vi "onProcessStart.vi"(8 "error in (no error)":errorcluster, 11 "SystemController":refnum<class "SystemController.lvclass">) -> (0 "error out":errorcluster, 3 "SystemController out":refnum<class "SystemController.lvclass">)   [LabVIEW 2017, in "SystemController.lvclass"]
doc: "JKI State Machine Objects (SMO) 1.3.0.56\nJKI - JKI\nCopyright (c) 2017, JKI"
uses:
  SystemController.lvclass
  Camera/Camera_IMAQdx_class/Camera_IMAQdx.lvclass
  C:/VIT/simpleImageProcessingExample/lv_src/Camera/Camera_class/Camera.lvclass
  Camera/Camera_Sim_class/Camera_Sim.lvclass
  <vilib>/JKI/JKI SMO/SMO/SMO.lvclass
  ImageFacialDetection_class/ImageFacialDetection.lvclass
  Camera/Camera_class/Camera.lvclass
panel:
  # "For instructions on how to use the JKI State Machine Objects, examples and video tutorials, visit:\nhttp://jki.net/state-machine-objects/\n\nJKI State Machine Objects™\nhttp://jki.net/state-machine-objects/\nCopyright (C) 2005-2015, JKI <info@jki.net>\nALL RIGHTS RESERVED"
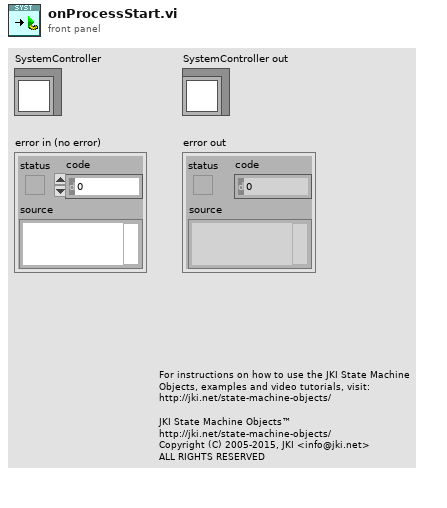
[diagram p1: front panel]
types:
  T1 = typedef "SystemController.lvclass/Configuration--Cluster.ctl" = cluster{"Camera":T2, "Find Eyes":bool, "Acquisition Rate (ms)":i32, "Image Buffer Length":i32}
  T2 = typedef "SystemController.lvclass/CameraConfig--Cluster.ctl" = cluster{"Simulate Camera":bool, "IMAQ Camera":T3, "Simulated Image Folder":path}
  T3 = typedef "Camera_IMAQdx.lvclass/Configuration--Cluster.ctl" = cluster{"Camera Interface Name":string, "Number of Buffers":u32, "Image Name":string, "Image Type":T4}
  T4 = typedef "Image Type" = u32
  T5 = cluster{"reference out":refnum<class "Camera.lvclass">, "reference out":refnum<class "ImageFacialDetection.lvclass">}
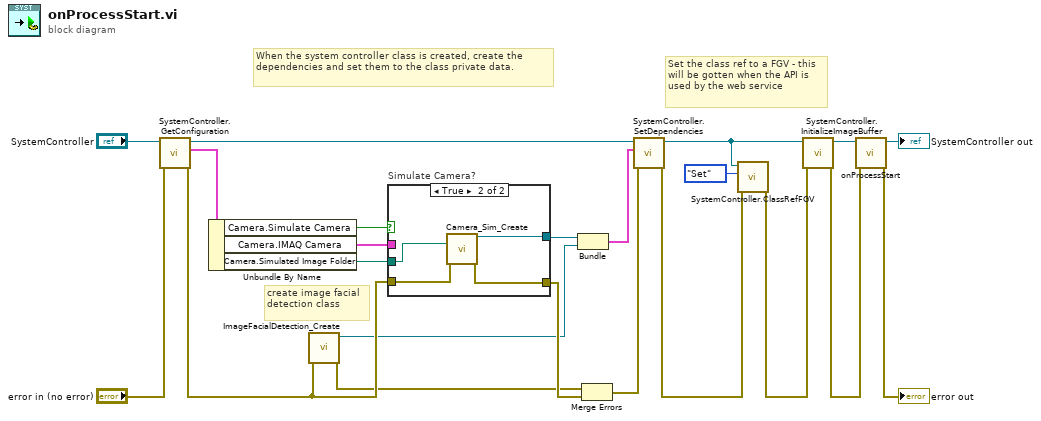
[diagram p0: block diagram]
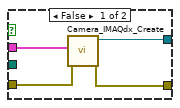
[diagram p2: hidden frame]
diagram:
  # "Set the class ref to a FGV - this will be gotten when the API is used by the web service"
  # "create image facial detection class"
  # "When the system controller class is created, create the dependencies and set them to the class private data."
  n1 = call "SystemController.GetConfiguration.vi"("error in (no error)"="error in (no error)", "SystemController"="SystemController") -> ("error out"=w10:errorcluster, "Configuration"=w17:T1, "SystemController out"=w19:refnum<class "SystemController.lvclass">)  [unwired: 7 in]
  n2 = Unbundle By Name(w17) -> ("Camera.Simulate Camera"=w16:bool, "Camera.IMAQ Camera"=w15:T3, "Camera.Simulated Image Folder"=w14:path)
  n3 = call "ImageFacialDetection_Create.vi"("error in (no error)"=w10) -> ("error out"=w8:errorcluster, "reference out"=w7:refnum<class "ImageFacialDetection.lvclass">)  [unwired: 9 in]
  n4 = case "Simulate Camera?" shown="True" w16 {
    tunnel: w15 -> [w26 _]
    tunnel: w14 -> [_ w30]
    tunnel: [w25 w29] -> w12
    tunnel: w10 -> [w24 w28]
    tunnel: [w23 w27] -> w13
    frame False {
      n5 = call "Camera_IMAQdx_Create.vi"("error in (no error)"=w24, "Configuration"=w26) -> ("error out"=w23:errorcluster, "reference out"=w25:refnum<class "Camera_IMAQdx.lvclass">)  [unwired: 8 in]
    }
    frame True {
      n6 = call "Camera_Sim_Create.vi"("Simulated Image Directory"=w30, "error in (no error)"=w28) -> ("reference out"=w29:refnum<class "Camera_Sim.lvclass">, "error out"=w27:errorcluster)  [unwired: 12 in]
    }
  }
  n7 = Bundle("reference out"=w12, "reference out"=w7) -> (w11:T5)  [unwired: 1 in]
  n8 = Merge Errors(w8, w13) -> (w9:errorcluster)
  n9 = call "SystemController.SetDependencies.vi"("error in (no error)"=w9, "Dependencies"=w11, "SystemController"=w19) -> ("error out"=w6:errorcluster, "SystemController out"=w4:refnum<class "SystemController.lvclass">)  [unwired: 7 in]
  n10 = call "SystemController.ClassRefFGV.vi"("error in (no error)"=w6, "Set/Get"=enum16{"Set", "Get"}."Set", "SystemController"=w4) -> ("error out"=w2:errorcluster)  [unwired: 7 in, 1 out]
  n11 = call "SystemController.InitializeImageBuffer.vi"("error in (no error)"=w2, "SystemController"=w4) -> ("error out"=w1:errorcluster, "SystemController out"=w3:refnum<class "SystemController.lvclass">)  [unwired: 8 in]
  n12 = call-parent "onProcessStart.vi"("error in (no error)"=w1, "SMO"=w3) -> ("error out"=→"error out":errorcluster, "SMO out"=→"SystemController out":refnum<class "SystemController.lvclass">)  [unwired: 8 in]
